vi "Gas Pump Test.vi"(8 "error in":errorcluster, 9 "Test Results In":T9, 11 "PAS In":T1) -> (0 "error out":errorcluster, 1 "Test Results Out":T9, 3 "Session Handle out":T1, 5 "Pass":bool)   [LabVIEW 2015]
uses:
  Controls/Test Results.ctl
  Controls/Step Result.ctl
  Controls/Startup Test.ctl
  Controls/Test Information.ctl
  Controls/Vacuum Test.ctl
  Controls/Test Timing.ctl
  Controls/Vaccum Thresholds.ctl
  Controls/Helium Test.ctl
  Controls/Helium Thresholds.ctl
  Controls/Startup Thresholds.ctl
  CAN Communication/Oil/Typedefs/Session Handle.ctl
  CAN Communication/Oil/Oil.lvclass
  User Interface/UI Handler/UI Handler.lvclass
panel:
  out "Test Configuration Out":T2
  in  "Test Configuration In":T2
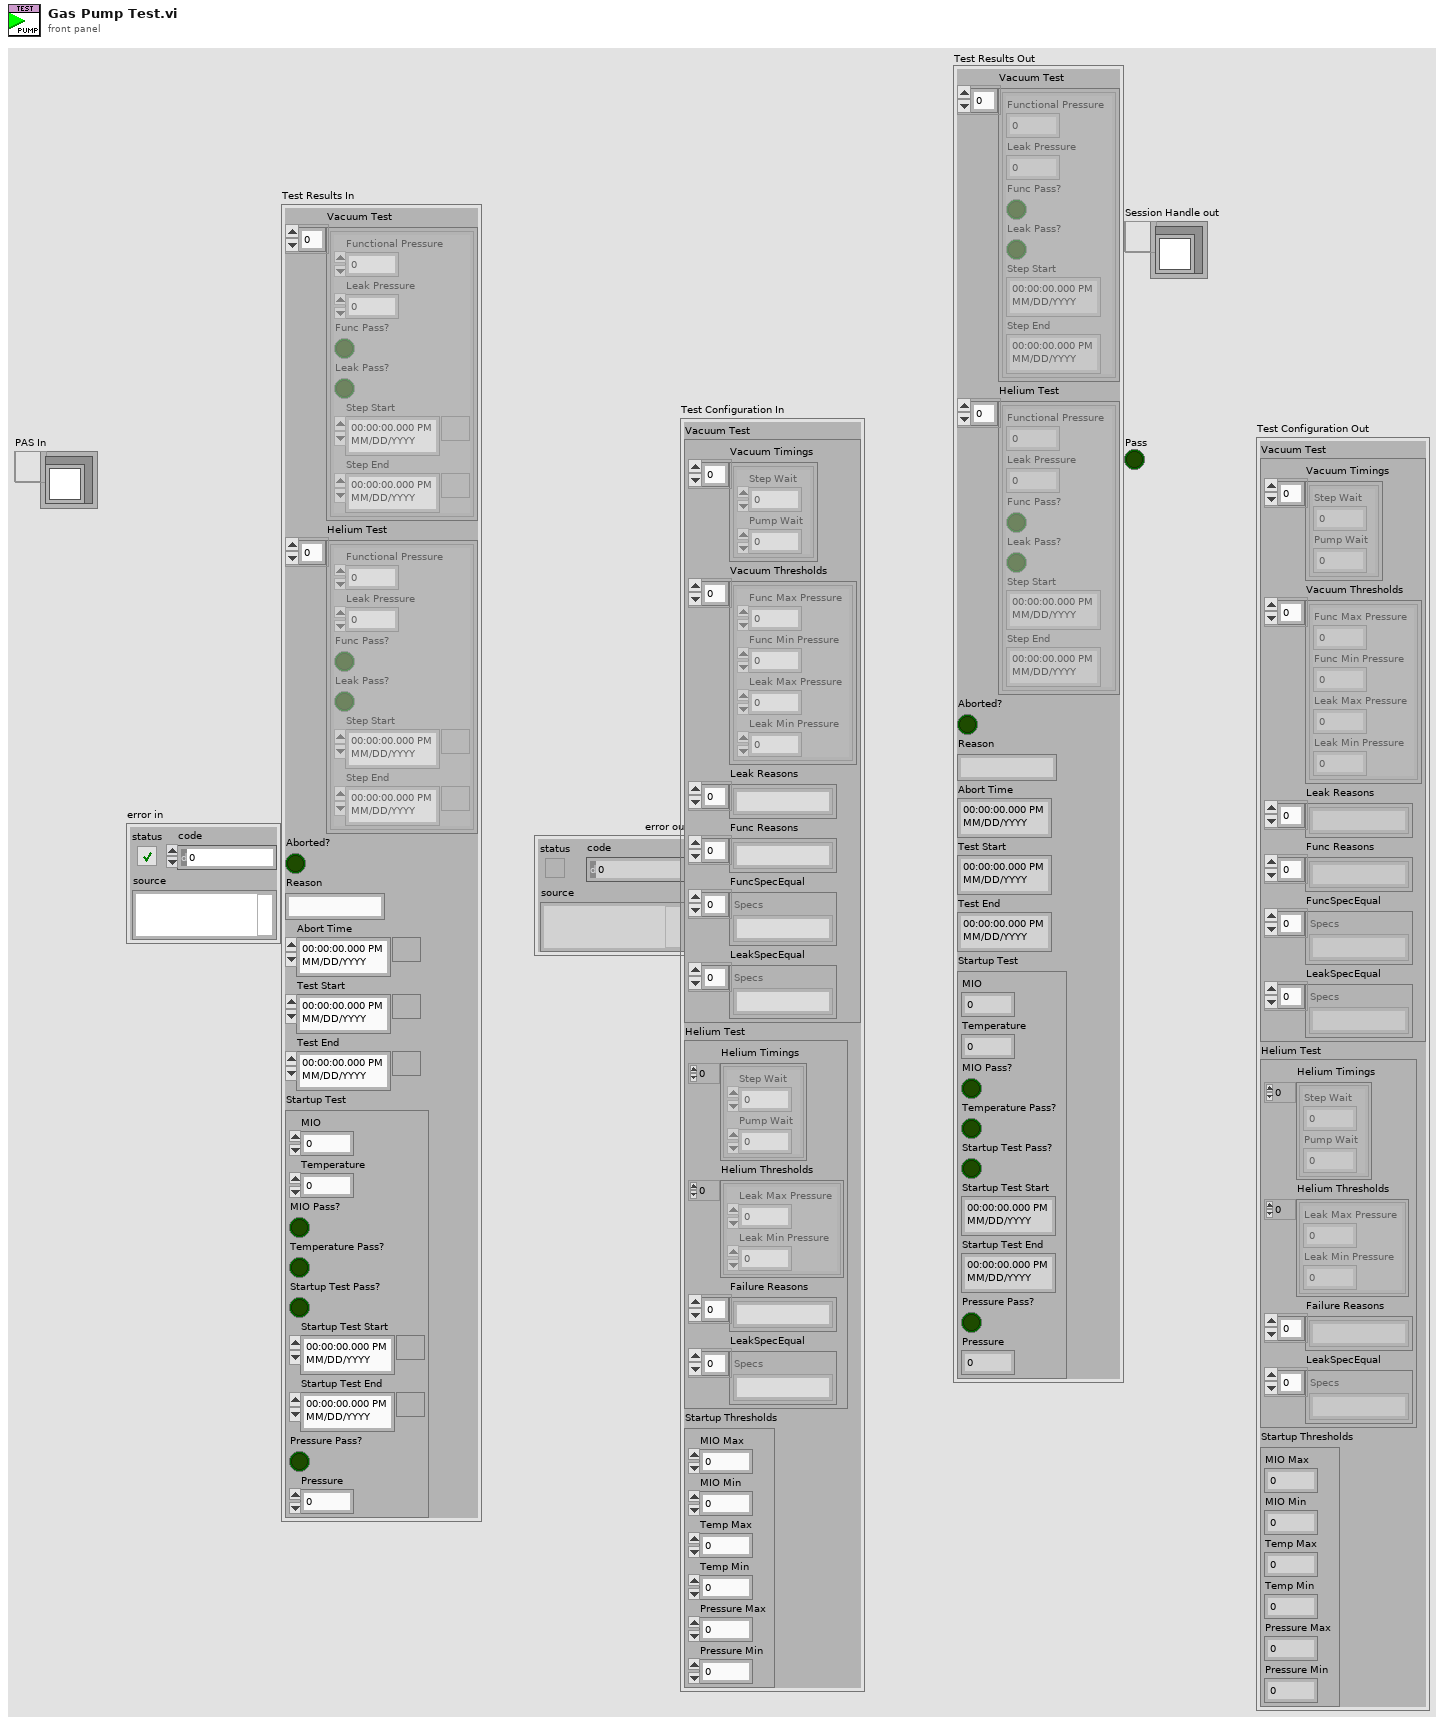
[diagram p1: front panel]
types:
  T1 = typedef "Oil.lvclass/Session Handle.ctl" = refnum<data-value>
  T2 = typedef "Test Information.ctl" = cluster{"Vacuum Test":T3, "Helium Test":T6, "Startup Thresholds":T8}
  T3 = typedef "Vacuum Test.ctl" = cluster{"Vacuum Timings":T4[], "Vacuum Thresholds":T5[], "Leak Reasons":string[], "Func Reasons":string[], "FuncSpecEqual":string[], "LeakSpecEqual":string[]}
  T4 = typedef "Test Timing.ctl" = cluster{"Step Wait":dbl, "Pump Wait":dbl}
  T5 = typedef "Vaccum Thresholds.ctl" = cluster{"Func Max Pressure":dbl, "Func Min Pressure":dbl, "Leak Max Pressure":dbl, "Leak Min Pressure":dbl}
  T6 = typedef "Helium Test.ctl" = cluster{"Helium Timings":T4[], "Helium Thresholds":T7[], "Failure Reasons":string[], "LeakSpecEqual":string[]}
  T7 = typedef "Helium Thresholds.ctl" = cluster{"Leak Max Pressure":dbl, "Leak Min Pressure":dbl}
  T8 = typedef "Startup Thresholds.ctl" = cluster{"MIO Max":dbl, "MIO Min":dbl, "Temp Max":dbl, "Temp Min":dbl, "Pressure Max":dbl, "Pressure Min":dbl}
  T9 = typedef "Test Results.ctl" = cluster{"Vacuum Test":T10[], "Helium Test":T10[], "Aborted?":bool, "Reason":string, "Abort Time":timestamp, "Test Start":timestamp, "Test End":timestamp, "Startup Test":T11}
  T10 = typedef "Step Result.ctl" = cluster{"Functional Pressure":dbl, "Leak Pressure":dbl, "Func Pass?":bool, "Leak Pass?":bool, "Step Start":timestamp, "Step End":timestamp}
  T11 = typedef "Startup Test.ctl" = cluster{"MIO":dbl, "Temperature":dbl, "MIO Pass?":bool, "Temperature Pass?":bool, "Startup Test Pass?":bool, "Startup Test Start":timestamp, "Startup Test End":timestamp, "Pressure Pass?":bool, "Pressure":dbl}
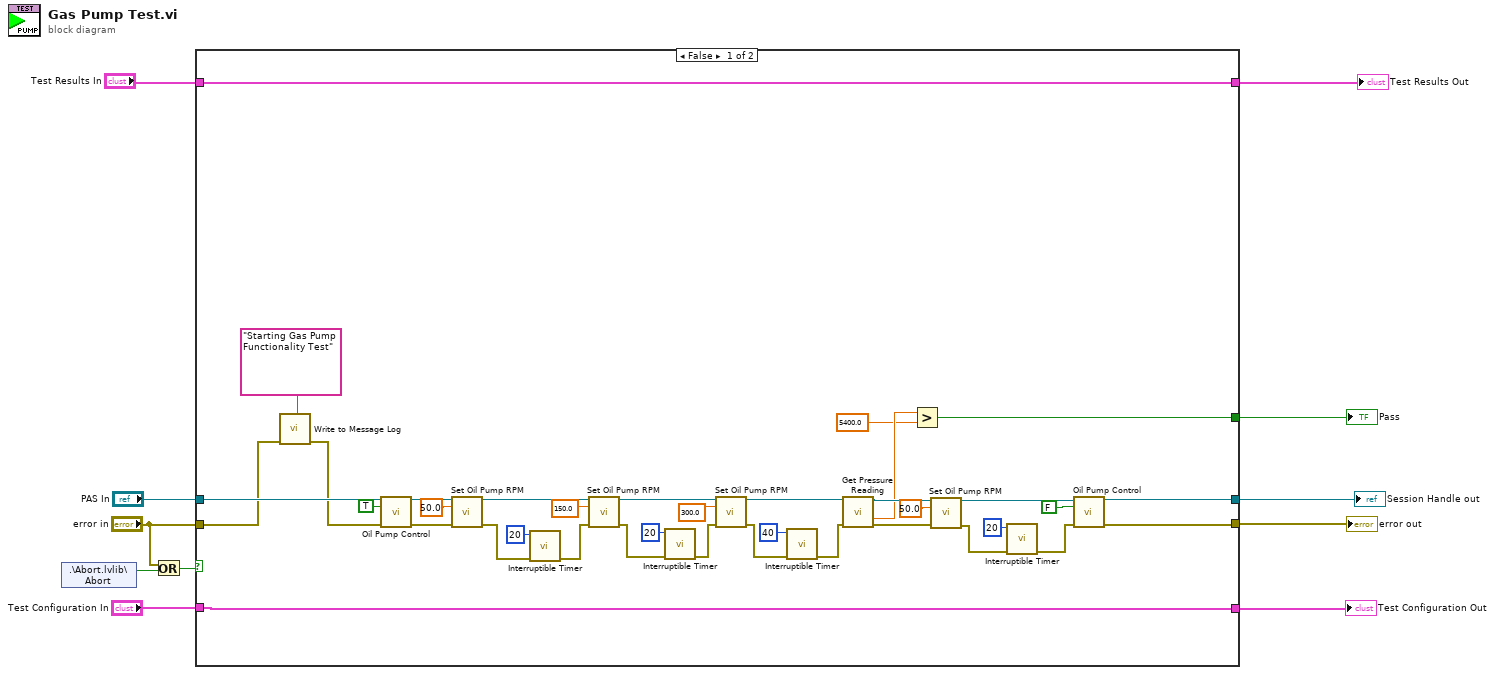
[diagram p0: block diagram]
diagram:
  n1 = shared-variable ".\\Abort.lvlib\\Abort"() -> (w5:bool)  [unwired: 1 in, 1 out]
  n2 = Or(x="error in", y=w5) -> (x .or. y?=w11:bool)
  n3 = case shown="False" w11 {
    tunnel: "error in" -> [w14 w50]
    tunnel: "Test Results In" -> [w47 w51]
    tunnel: [w47 w51] -> w10
    tunnel: [w16 w50] -> w9
    tunnel: "Test Configuration In" -> [w21 w49]
    tunnel: [w21 w49] -> w6
    tunnel: [w18 _] -> w3
    tunnel: "PAS In" -> [w17 _]
    tunnel: [w15 _] -> w1
    frame False {
      n4 = call "Write to Message Log.vi"("error in (no error)"=w14, "Message"="Starting Gas Pump Functionality Test") -> ("error out"=w13:errorcluster)  [unwired: 9 in]
      n5 = call "Oil Pump Control.vi"("Session Handle in"=w17, "On?"=TRUE, "error in (no error)"=w13) -> ("Session Handle out"=w46:T1, "error out"=w45:errorcluster)  [unwired: 9 in, 2 out]
      n6 = call "Set Oil Pump RPM.vi"("Session Handle in"=w46, "RPM"=50.0, "error in (no error)"=w45) -> ("Session Handle out"=w40:T1, "error out"=w42:errorcluster)  [unwired: 9 in, 2 out]
      n7 = call "Interruptible Timer.vi"("error in (no error)"=w42, "Wait (s)"=20) -> ("error out"=w41:errorcluster)  [unwired: 7 in, 2 out]
      n8 = call "Set Oil Pump RPM.vi"("Session Handle in"=w40, "RPM"=150.0, "error in (no error)"=w41) -> ("Session Handle out"=w35:T1, "error out"=w37:errorcluster)  [unwired: 9 in, 2 out]
      n9 = call "Interruptible Timer.vi"("error in (no error)"=w37, "Wait (s)"=20) -> ("error out"=w34:errorcluster)  [unwired: 7 in, 2 out]
      n10 = call "Set Oil Pump RPM.vi"("Session Handle in"=w35, "RPM"=300.0, "error in (no error)"=w34) -> ("Session Handle out"=w29:T1, "error out"=w33:errorcluster)  [unwired: 9 in, 2 out]
      n11 = call "Interruptible Timer.vi"("error in (no error)"=w33, "Wait (s)"=40) -> ("error out"=w30:errorcluster)  [unwired: 7 in, 2 out]
      n12 = call "Get Pressure Reading.vi"("Session Handle in"=w29, "error in (no error)"=w30) -> ("Session Handle out"=w27:T1, "Pressure"=w20:dbl, "error out"=w26:errorcluster)  [unwired: 10 in, 1 out]
      n13 = Greater?(x=w20, y=5400.0) -> (0:w18:bool)
      n14 = call "Set Oil Pump RPM.vi"("Session Handle in"=w27, "RPM"=50.0, "error in (no error)"=w26) -> ("Session Handle out"=w23:T1, "error out"=w24:errorcluster)  [unwired: 9 in, 2 out]
      n15 = call "Interruptible Timer.vi"("error in (no error)"=w24, "Wait (s)"=20) -> ("error out"=w22:errorcluster)  [unwired: 7 in, 2 out]
      n16 = call "Oil Pump Control.vi"("Session Handle in"=w23, "On?"=FALSE, "error in (no error)"=w22) -> ("Session Handle out"=w15:T1, "error out"=w16:errorcluster)  [unwired: 9 in, 2 out]
    }
    frame True {
    }
  }
  "error out" <- w9
  "Test Results Out" <- w10
  "Test Configuration Out" <- w6
  "Pass" <- w3
  "Session Handle out" <- w1
